vi "Find Module Virtual Folder.vi"(8 "error in":errorcluster, 10 "Virtual Folder":string, 11 "Children":refnum<vi>[](array[refnum])) -> (0 "error out":errorcluster, 2 "Found?":bool, 3 "ProjectItem out":refnum<vi>)   [LabVIEW 2020, in "ConstantErrorsMaker.lvlib"]
uses:
  ConstantErrorsMaker.lvlib
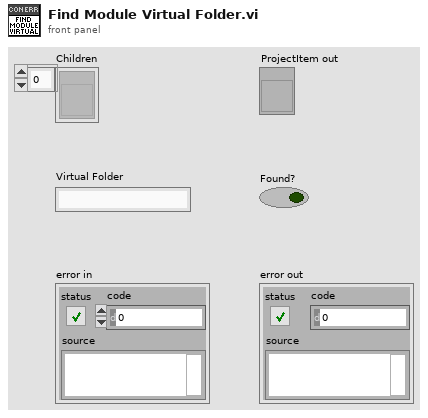
[diagram p1: front panel]
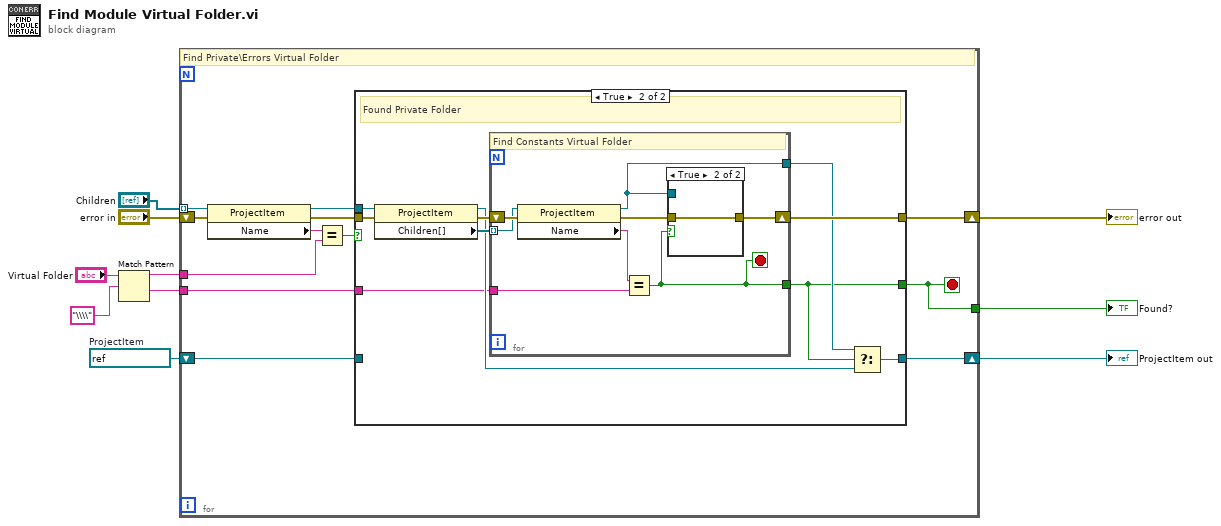
[diagram p0: block diagram]
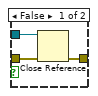
[diagram p3: hidden frame]
diagram:
  w2 = refnum<vi> refnum  # ProjectItem
  n1 = Match Pattern(string="Virtual Folder", regular expression="\\\\") -> (before substring=w6:string, after substring=w5:string)  [unwired: 1 in, 2 out]
  n2 = for {
    tunnel: "Children" -> [w19] mode=indexing
    shift-right: [w20] -> w10
    shift-left: "error in" -> [w22]
    tunnel: w6 -> [w14]
    tunnel: w5 -> [w13]
    shift-right: [w15] -> w3
    shift-left: w2 -> [w12]
    tunnel: [w11] -> w1
    stop <- w11 stop-if-true
    # "Find Private\\Errors Virtual Folder"
    n3 = property class="ProjectItem"(reference=w19, error in=w22) -> (reference out=w17:refnum<vi>, error out=w21:errorcluster, "Name"=w18:string)
    n4 = Equal?(x=w18, y=w14) -> (x = y?=w16:bool)
    n5 = case shown="True" w16 {
      tunnel: w21 -> [w24 w34]
      tunnel: [w24 w32] -> w20
      tunnel: w17 -> [_ w31]
      tunnel: [_ w25] -> w11
      tunnel: [w23 w27] -> w15
      tunnel: w13 -> [_ w26]
      tunnel: w12 -> [w23 _]
      frame False {
      }
      frame True {
        # "Found Private Folder"
        n6 = property class="ProjectItem"(reference=w31, error in=w34) -> (reference out=w28:refnum<vi>, error out=w33:errorcluster, "Children[]"=w30:refnum<vi>[])
        n7 = for {
          tunnel: w30 -> [w39] mode=indexing
          tunnel: [w37] -> w25
          shift-right: [w40] -> w32
          shift-left: w33 -> [w42]
          tunnel: [w36] -> w29
          tunnel: w26 -> [w35]
          stop <- w37 stop-if-true
          # "Find Constants Virtual Folder"
          n8 = property class="ProjectItem"(reference=w39, error in=w42) -> (reference out=w36:refnum<vi>, error out=w41:errorcluster, "Name"=w38:string)
          n9 = Equal?(x=w38, y=w35) -> (x = y?=w37:bool)
          n10 = case shown="True" w37 {
            tunnel: w41 -> [w45 w46]
            tunnel: [w44 w46] -> w40
            tunnel: w36 -> [w43 _]
            frame False {
              n11 = Close Reference(reference=w43, error in (no error)=w45) -> (error out=w44:errorcluster)
            }
            frame True {
            }
          }
        }
        n12 = Select(t=w29, s=w25, f=w28) -> (s? t:f=w27:refnum<vi>)
      }
    }
  }
  "Found?" <- w1
  "ProjectItem out" <- w3
  "error out" <- w10
